vi "Global_HW_Data Out.vi"() -> ()   [LabVIEW 2017, in "TemplateActuator.lvlib"]
uses:
  TemplateActuator.lvlib
  Cluster_HW Status.ctl
panel:
  in  "HW_Actuator_Status":T1
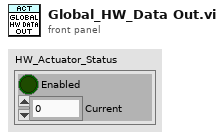
[diagram p1: front panel]
types:
  T1 = typedef "TemplateActuator.lvlib/Cluster_HW Status.ctl" = cluster{"Enabled":bool, "Current":dbl}
diagram:
